vi "Lightfield_Cam1.vi"() -> ()   [LabVIEW 2018]
uses:
  <vilib>/Enthought/Python Integration Toolkit/api/Console Visibility.ctl
  Global Variables.vi
  ProgramData/Documents/Princeton Instruments/LightField/Add-in and Automation SDK/Samples/LabVIEW Automation/lightfield-automation-labview/LightField Automation.lvclass
  <vilib>/Enthought/Python Integration Toolkit/Python Integration Toolkit.lvlib
panel:
  in  "Logfile?":bool
  in  "Experiment Name":string="TestCamera"
  in  "File Path":path=path "C:/Labview Test Data/2018-10-09/UnspecifiedProj/Temp Dependence/PI_Cam1_400C"
  in  "stop":bool
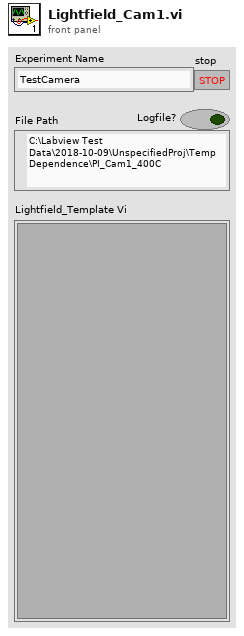
[diagram p1: front panel]
types:
  T1 = typedef "Python Integration Toolkit.lvlib/Console Visibility.ctl" = enum16{"Show Console", "Show Console While Running", "Hide Console"}
  T2 = enum32{"Bad", "Idle", "Run top level", "Running"}
  T3 = typedef "Python Integration Toolkit.lvlib/Session ID.ctl" = u64
  T4 = cluster{"Project":u16, "SubFolder":string, "Filename (Meas. Description)":string, "Measurement index":i32}
  T5 = typedef "Python Integration Toolkit.lvlib/Python Objects.ctl" = variant
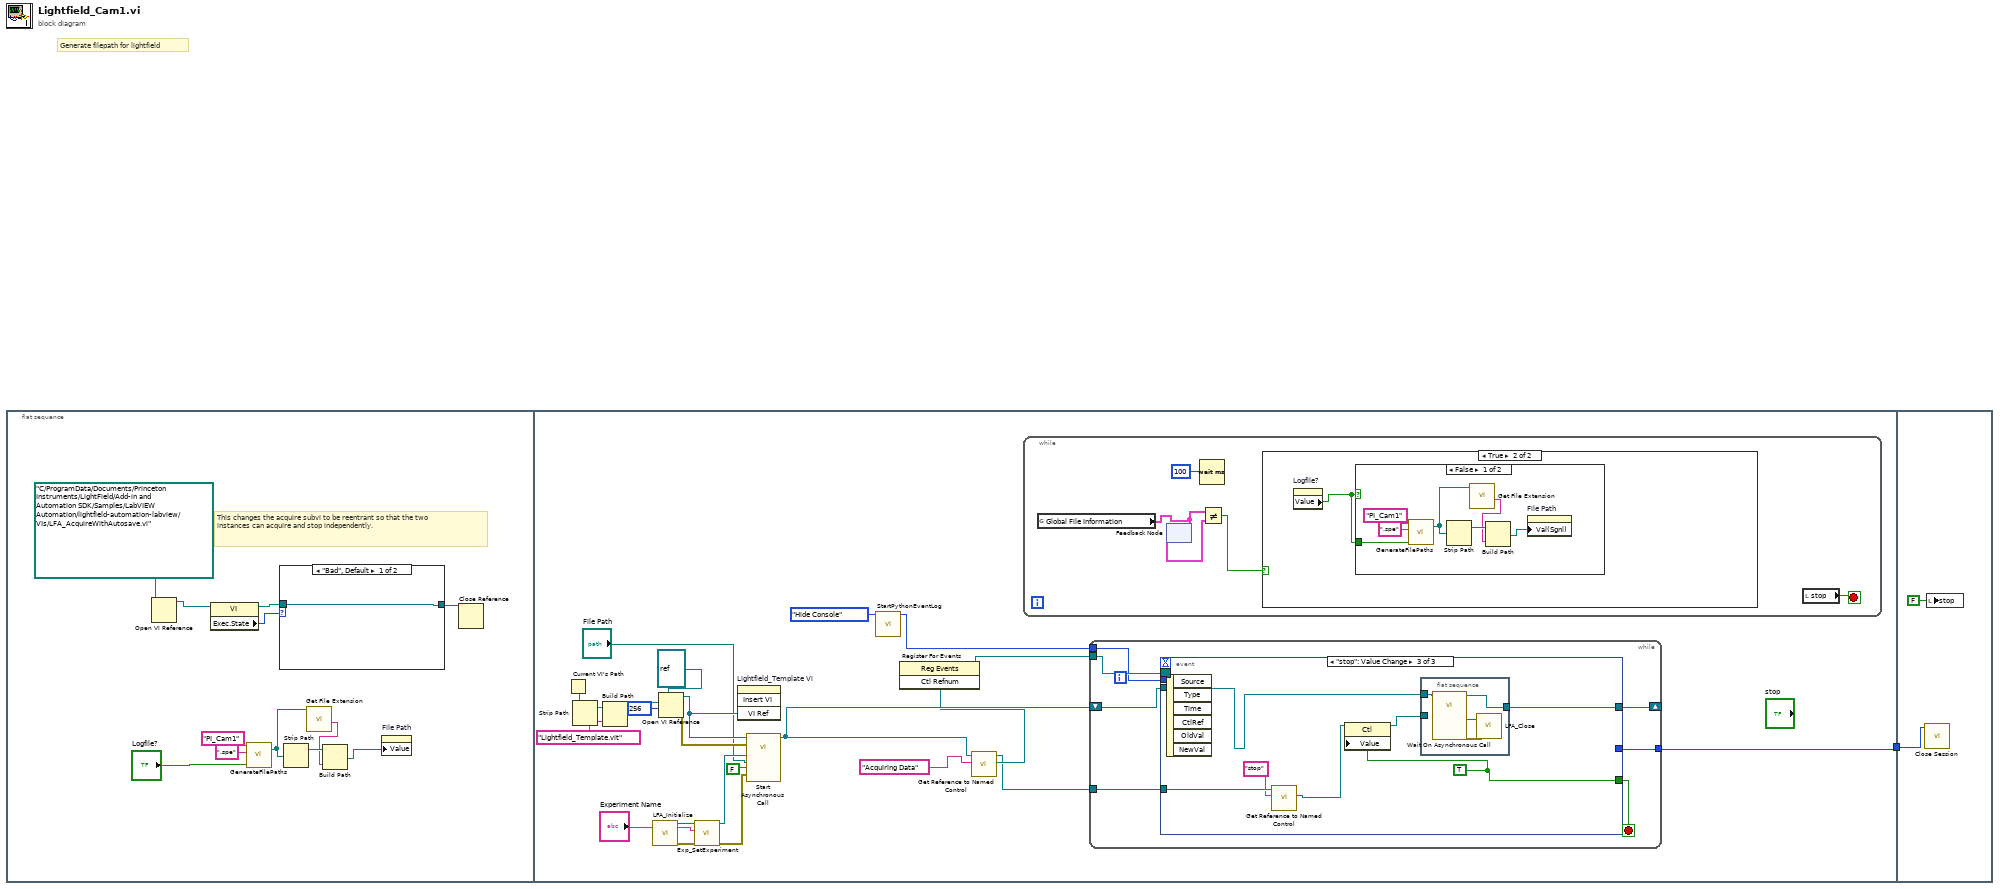
[diagram p0: block diagram]
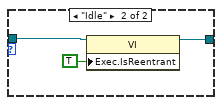
[diagram p2: hidden frame]
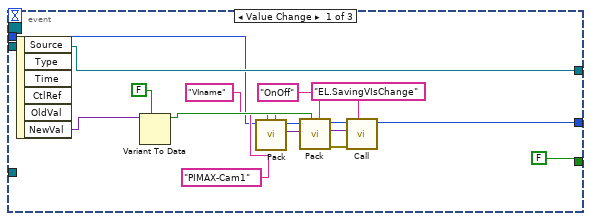
[diagram p5: hidden frame]
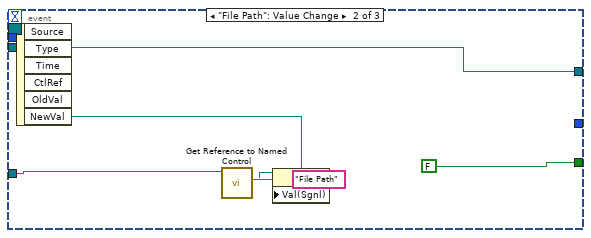
[diagram p6: hidden frame]
diagram:
  # "Generate filepath for lightfield"
  n1 = flat-sequence {
    tunnel: [w24] -> w1
    tunnel: w1 -> [w94]
    frame #0 {
      # "This changes the acquire subvi to be reentrant so that the two instances can acquire and stop independently."
      n2 = Open VI Reference(vi path=path "C:/ProgramData/Documents/Princeton Instruments/LightField/Add-in and Automation SDK/Samples/LabVIEW Automation/lightfield-automation-labview/VIs/LFA_AcquireWithAutosave.vi") -> (vi reference=w4:refnum<vi>)  [unwired: 5 in, 1 out]
      n3 = property class="VI"(reference=w4) -> (reference out=w2:refnum<vi>, "Exec.State"=w3:T2)  [unwired: 1 in, 1 out]
      n4 = call "GenerateFilePaths.vi"("Logfile?"="Logfile?", "Extension (.tdms)"=".spe" ("Extension"), "Device Name"="PI_Cam1" ("Instrument")) -> ("Path"=w8:path)  [unwired: 2 in]
      n5 = case shown="\"Bad\", Default" w3 {
        tunnel: [w14 w16] -> w11
        tunnel: w2 -> [w14 w15]
        frame "Bad", Default {
        }
        frame "Idle" {
          n6 = property class="VI"(reference=w15, "Exec.IsReentrant"=TRUE ("Execution:Is Reentrant")) -> (reference out=w16:refnum<vi>)  [unwired: 1 in, 1 out]
        }
      }
      n7 = Strip Path(path=w8) -> (stripped path=w7:path)  [unwired: 1 out]
      n8 = call <vilib>:"Get File Extension.vi"("file"=w8) -> ("filename without extension"=w6:string)  [unwired: 6 in, 4 out]
      n9 = Build Path(base path=w7, name or relative path=w6) -> (appended path=w5:path)
      n10 = property on="File Path" class="Path"("Value"=w5) -> ()  [unwired: 2 in, 2 out]
      n11 = Close Reference(reference=w11) -> ()  [unwired: 1 in, 1 out]
    }
    frame #1 {
      n12 = Current VI's Path() -> (path=w37:path)
      n13 = Strip Path(path=w37) -> (stripped path=w38:path)  [unwired: 1 out]
      n14 = Build Path(base path=w38, name or relative path="Lightfield_Template.vit") -> (appended path=w34:path)
      n15 = call "LFA_Initialize.vi"() -> ("error out"=w40:errorcluster, "LightField Automation out"=w39:refnum<class "LightField Automation.lvclass">)  [unwired: 10 in]
      n16 = Open VI Reference(type specifier VI Refnum (for type only)=refnum<vi> refnum, vi path=w34, options=256) -> (vi reference=w32:refnum<vi>, error out=w31:errorcluster)  [unwired: 1 in, 2 out]
      n17 = call "Exp_SetExperiment.vi"("error in (no error)"=w40, "ExperimentName"="Experiment Name", "LightField Automation in"=w39) -> ("error out"=w30:errorcluster, "LightField Automation out"=w29:refnum<class "LightField Automation.lvclass">)  [unwired: 7 in]
      n18 = invoke on="Lightfield_Template Vi" class="SubPnl" method="Insert VI"("VI Ref"=w32) -> ()  [unwired: 3 in, 4 out]
      n19 = call-by-ref "Start Asynchronous Call"(reference=w32, error in=w31, "error out"=w30, "Single Run"=FALSE, "Filepath"="File Path", "LightField Automation in"=w29) -> (reference out=w23:refnum<vi>)  [unwired: 6 in, 3 out]
      n20 = call "StartPythonEventLog.vi"("Console Visibility"=Console_Visibility."Hide Console") -> ("Session ID out"=w25:T3)  [unwired: 10 in]
      n21 = call "Get Reference to Named Control.vi"("Control Name"="Acquiring Data" ("element"), "Front Panel Ref"=w23) -> ("Ctl Refnum"=w21:refnum<vi>, "Panel Ref Out"=w20:refnum<vi>)  [unwired: 7 in, 1 out]
      n22 = register-events(w21) -> (reference out=w26:refnum<event-registration>)  [unwired: 2 in, 1 out]
      n23 = while {
        stop <- w45 stop-if-true
        n24 = global read "Global Variables.vi" "Global File Information"() -> (w43:T4)
        n25 = feedback #1() -> (w42:T4)  [unwired: 1 in]
        n26 = feedback-in #1(w43) -> ()
        n27 = Wait (ms)(milliseconds to wait=100) -> ()  [unwired: 1 out]
        n28 = Not Equal?(x=w43, y=w42) -> (x != y?=w41:bool)
        n29 = case shown="True" w41 {
          frame False {
          }
          frame True {
            n30 = property on="Logfile?" class="Bool (strict)"() -> ("Value"=w46:bool)  [unwired: 2 in, 2 out]
            n31 = case shown="False" w46 {
              tunnel: w46 -> [w48 _]
              frame False {
                n32 = call "GenerateFilePaths.vi"("Logfile?"=w48, "Extension (.tdms)"=".spe" ("Extension"), "Device Name"="PI_Cam1" ("Instrument")) -> ("Path"=w51:path)  [unwired: 2 in]
                n33 = Strip Path(path=w51) -> (stripped path=w50:path)  [unwired: 1 out]
                n34 = call <vilib>:"Get File Extension.vi"("file"=w51) -> ("filename without extension"=w49:string)  [unwired: 6 in, 4 out]
                n35 = Build Path(base path=w50, name or relative path=w49) -> (appended path=w47:path)
                n36 = property on="File Path" class="Path"("Val(Sgnl)"=w47) -> ()  [unwired: 2 in, 2 out]
              }
              frame True {
              }
            }
          }
        }
        n37 = local read "stop"() -> (w45:bool)
      }
      n38 = while {
        shift-right: [w58] -> _
        shift-left: w23 -> [w59]
        tunnel: w26 -> [w57]
        tunnel: w25 -> [w56]
        tunnel: [w55] -> w24
        tunnel: w20 -> [w54]
        stop <- w60 stop-if-true
        n39 = event shown="[2] \"stop\": Value Change" {
          selector: w57 -> [_ _ _]
          dyn-events: _ -> [_ _ _]
          timeout: _ -> [_ _ _]
          tunnel: [FALSE FALSE w89] -> w60
          tunnel: w59 -> [w75 w80 w88]
          tunnel: [w75 w80 w87] -> w58
          tunnel: w56 -> [w68 _ _]
          tunnel: [w61 _ _] -> w55
          tunnel: w54 -> [_ w78 w85]
          event Value Change {
            n40 = event-data() -> ("NewVal"=w74:variant)  [unwired: 1 in, 5 out]
            n41 = Variant To Data(type=FALSE, Variant=w74) -> (data=w72:bool)  [unwired: 1 in, 1 out]
            n42 = call <vilib>:"Pack.vi"("Keyword Name"="VIname", "Argument"="PIMAX-Cam1", "Session ID"=w68) -> ("Python Object References Out"=w63:T5, "Session ID out"=w67:T3)  [unwired: 6 in, 1 out]
            n43 = call <vilib>:"Pack.vi"("Keyword Name"="OnOff", "Argument"=w72, "Python Object References In"=w63, "Session ID"=w67) -> ("error out"=w66:errorcluster, "Python Object References Out"=w65:T5, "Session ID out"=w64:T3)  [unwired: 5 in]
            n44 = call <vilib>:"Call.vi"("Function or Method Name"="EL.SavingVIsChange", "error in (no error)"=w66, "Python Object References In"=w65, "Session ID"=w64) -> ("Session ID out"=w61:T3)  [unwired: 5 in, 2 out]
          }
          event "File Path": Value Change {
            n45 = event-data() -> ("NewVal"=w82:path)  [unwired: 1 in, 5 out]
            n46 = call "Get Reference to Named Control.vi"("Control Name"="File Path" ("element"), "Front Panel Ref"=w78) -> ("Ctl Refnum"=w77:refnum<vi>)  [unwired: 7 in, 2 out]
            n47 = property class="Ctl"(reference=w77, "Val(Sgnl)"=w82) -> ()  [unwired: 1 in, 2 out]
          }
          event "stop": Value Change {
            w89 = TRUE
            n48 = event-data() -> ()  [unwired: 1 in, 6 out]
            n49 = call "Get Reference to Named Control.vi"("Control Name"="stop", "Front Panel Ref"=w85) -> ("Ctl Refnum"=w83:refnum<vi>)  [unwired: 7 in, 2 out]
            n50 = property class="Ctl"(reference=w83, "Value"=w89) -> (reference out=w86:refnum<vi>)  [unwired: 1 in, 1 out]
            n51 = flat-sequence {
              tunnel: w88 -> [w93]
              tunnel: w86 -> [_]
              tunnel: [w90] -> w87
              frame #0 {
                n52 = call-by-ref "Wait On Asynchronous Call"(reference=w93) -> (reference out=w90:refnum<vi>, "error out 2"=w91:errorcluster, "LightField Automation out"=w92:refnum<class "LightField Automation.lvclass">)  [unwired: 11 in, 1 out]
                n53 = call "LFA_Close.vi"("error in (no error)"=w91, "LightField Automation in"=w92) -> ()  [unwired: 8 in, 2 out]
              }
            }
          }
        }
      }
    }
    frame #2 {
      n54 = call <vilib>:"Close Session.vi"("Session ID"=w94) -> ()  [unwired: 10 in, 1 out]
      n55 = local write "stop"(FALSE ("stop")) -> ()
    }
  }
